vi "C State.vi"(0 "State":string, 1 "Front Leg PS":bool, 4 "Back Leg Up":bool, 5 "Mid Leg PS":bool, 6 "Back Leg PS":bool, 7 "Mid Leg Up":bool, 10 "Front Leg Up":bool, 11 "Back Claws Cmd":bool=TRUE, 13 "Front Claw Cmd":bool=TRUE) -> (20 "newState":string, 21 "Front Leg Cmd":enum16{"Down Closed", "Down Opened", "Up"}(ring), 22 "Drive Motor Enabled":bool=TRUE, 23 "Mid Leg Cmd":enum16{"Down Closed", "Down Opened", "Up"}(ring), 25 "Engage Back Leg":bool, 26 "Skids":bool)   [LabVIEW 2012]
uses:
  <vilib>/Rock Robotics/WPI/DriverStation/DriverStationLCD/WPI_DriverStationLCDLCDLine.ctl
  Begin/Global Variables.vi
panel:
  out "Error Text":string
  out "Console Msg":string
  out "Short Time Elapsed":bool caption="Time has Elapsed"
  out "Long Time Elapsed":bool
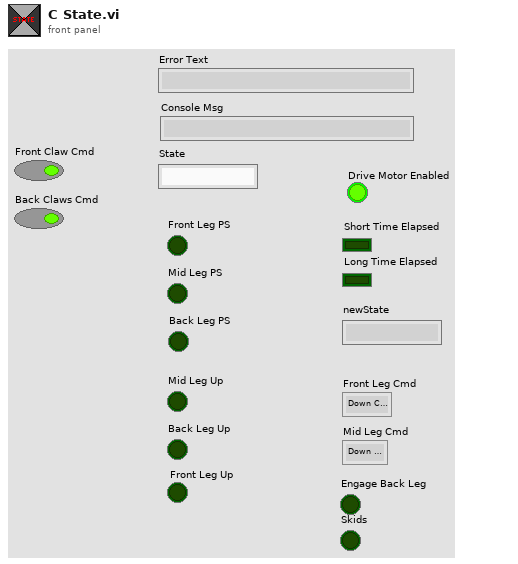
[diagram p1: front panel]
types:
  T1 = typedef "WPI_DriverStationLCDLCDLine.ctl" = enum16{"Main - Line 1", "User - Line 2", "User - Line 3", "User - Line 4", "User - Line 5", "User - Line 6"}
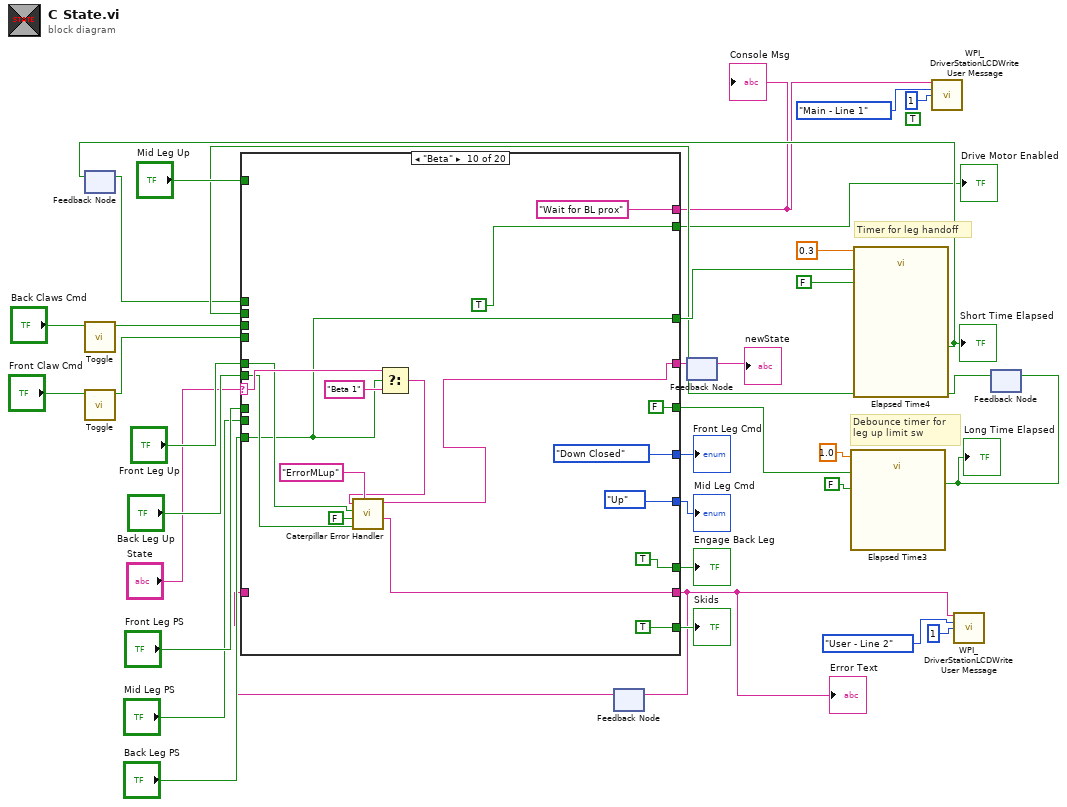
[diagram p0: block diagram]
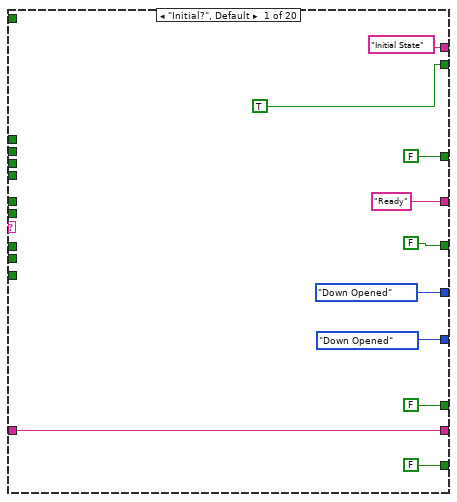
[diagram p2: hidden frame]
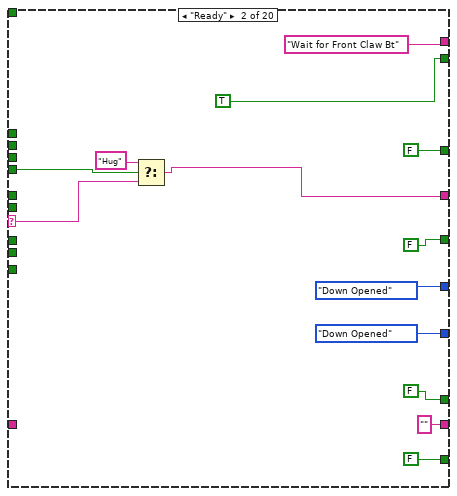
[diagram p3: hidden frame]
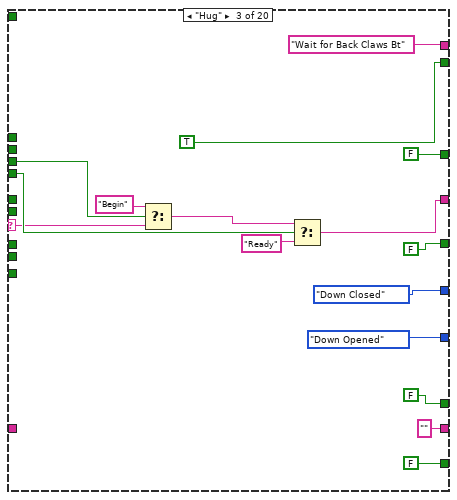
[diagram p4: hidden frame]
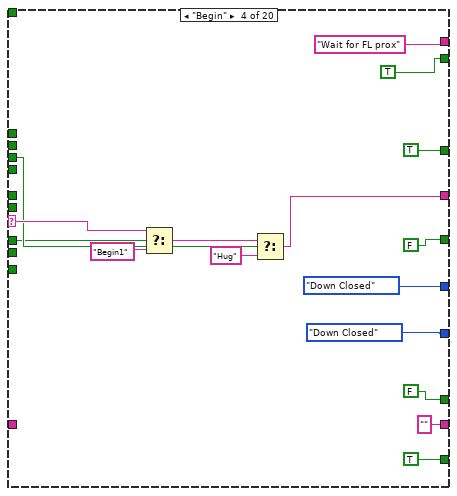
[diagram p5: hidden frame]
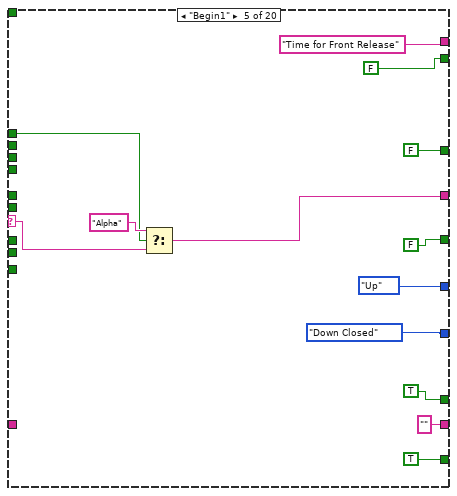
[diagram p6: hidden frame]
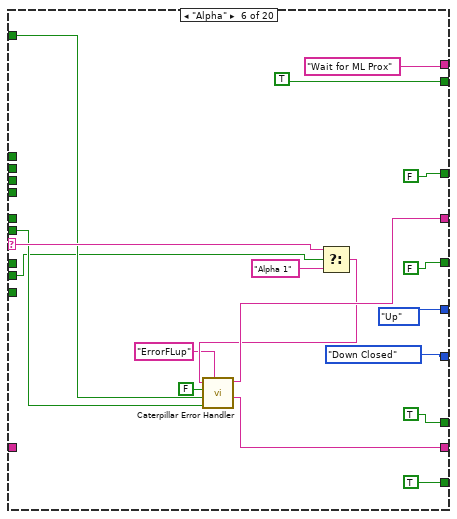
[diagram p7: hidden frame]
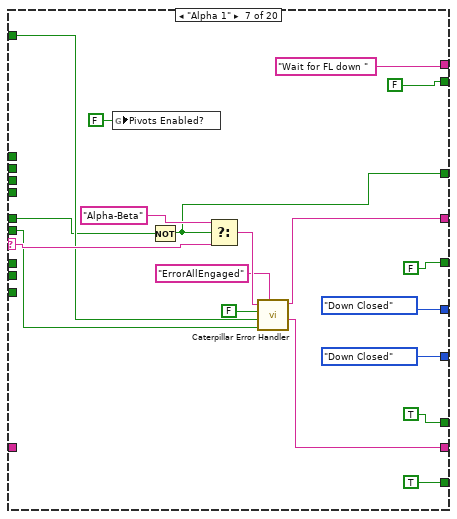
[diagram p8: hidden frame]
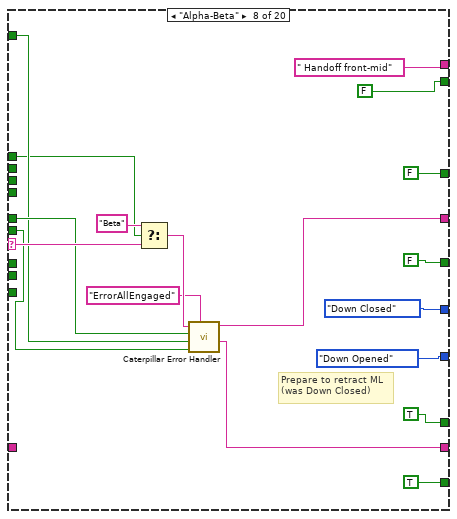
[diagram p9: hidden frame]
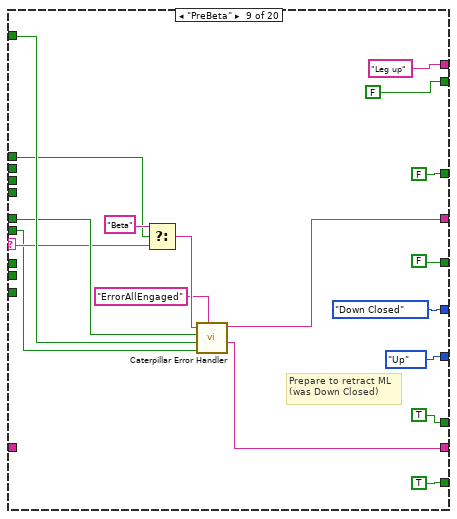
[diagram p10: hidden frame]
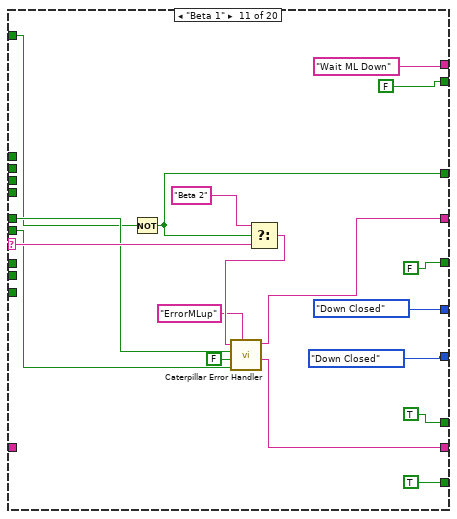
[diagram p11: hidden frame]
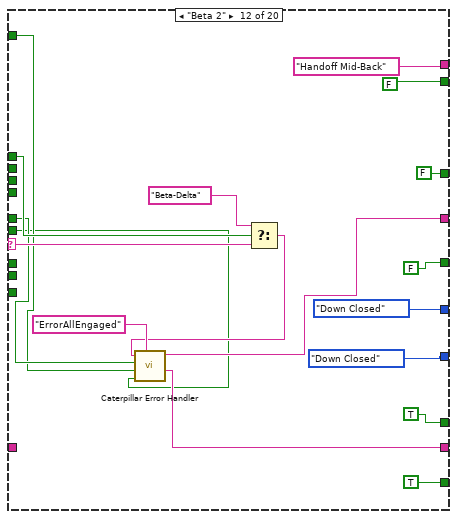
[diagram p12: hidden frame]
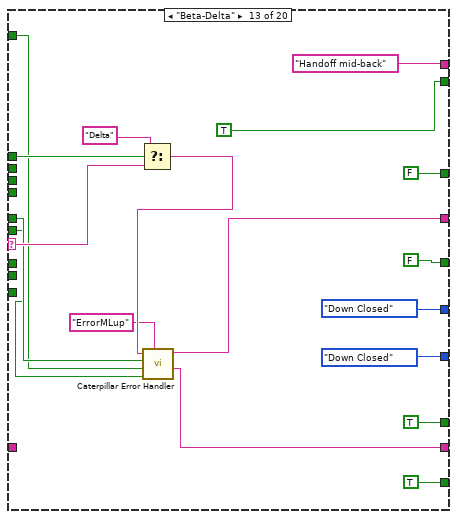
[diagram p13: hidden frame]
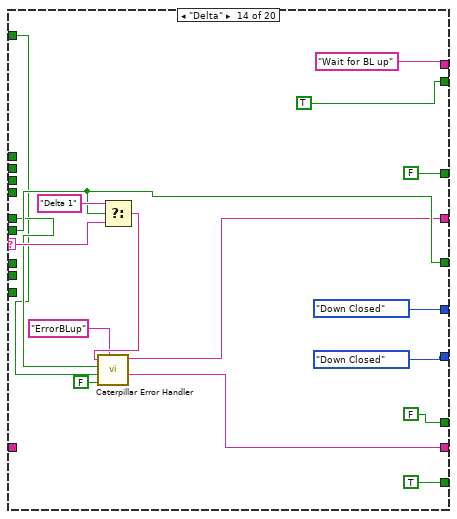
[diagram p14: hidden frame]
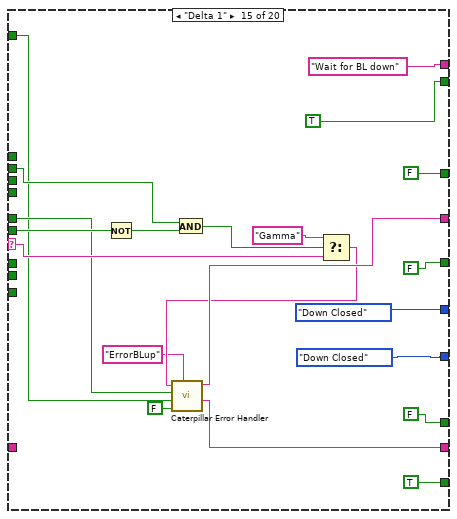
[diagram p15: hidden frame]
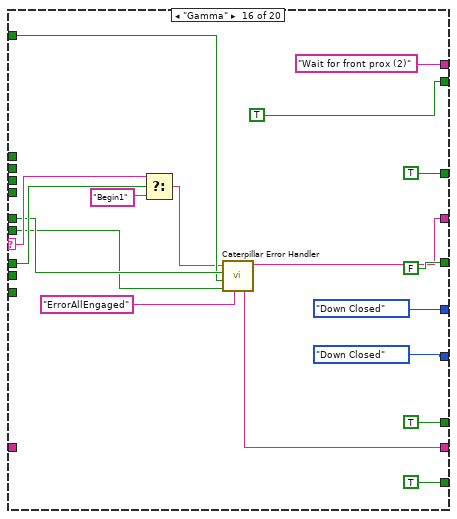
[diagram p16: hidden frame]
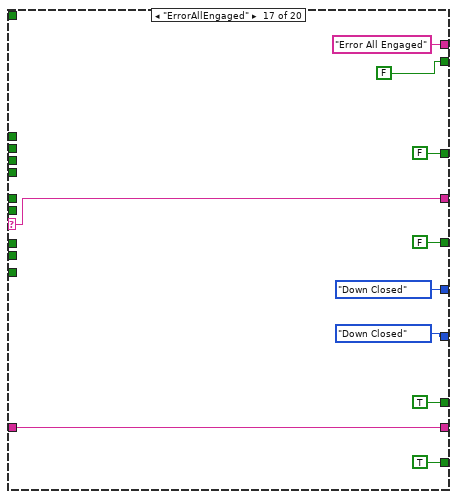
[diagram p17: hidden frame]
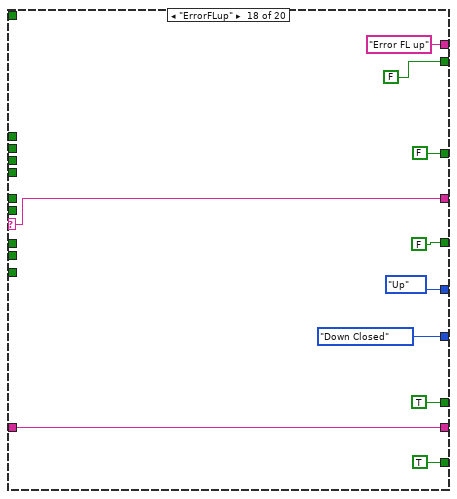
[diagram p18: hidden frame]
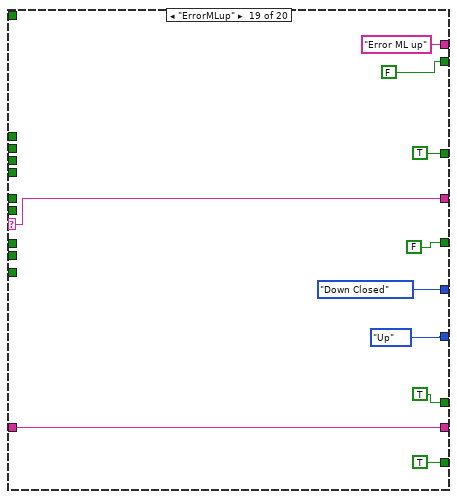
[diagram p19: hidden frame]
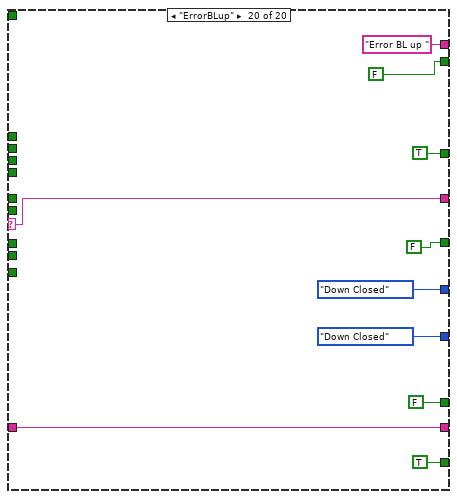
[diagram p20: hidden frame]
diagram:
  (unwired) TRUE ("clear line before write (T)")
  # "Timer for leg handoff"
  # "Debounce timer for \nleg up limit sw"
  n1 = feedback #1() -> (w17:bool)  [unwired: 1 in]
  n2 = call "Toggle.vi"("Boolean"="Back Claws Cmd") -> ("Toggled"=w15:bool)  [unwired: 10 in]
  n3 = call "Toggle.vi"("Boolean"="Front Claw Cmd") -> ("Toggled"=w24:bool)  [unwired: 10 in]
  n4 = feedback #2() -> (w6:string)  [unwired: 1 in]
  n5 = feedback #3() -> (→"newState":string)  [unwired: 1 in]
  n6 = feedback #4() -> (w23:bool)  [unwired: 1 in]
  n7 = case shown="\"Beta\"" "State" {
    selector: "State" -> [_ w56 w64 w84 w93 w119 w139 w156 w170 w186 w208 w226 w244 w260 w276 w301 w310 w320 w330 w340]
    tunnel: ["Ready" ("t") w49 w61 w78 w94 w111 w131 w150 w161 w183 w202 w217 w236 w254 w271 w293 w310 w320 w330 w340] -> w3
    tunnel: "Mid Leg PS" -> [_ _ _ _ _ w104 _ _ _ _ _ _ _ _ _ _ _ _ _ _]
    tunnel: "Front Leg PS" -> [_ _ _ w75 _ _ _ _ _ _ _ _ _ _ _ w300 _ _ _ _]
    tunnel: "Mid Leg Up" -> [_ _ _ _ _ w108 w130 w146 w173 _ w197 w214 w232 w250 w267 w289 _ _ _ _]
    tunnel: "Back Leg Up" -> [_ _ _ _ _ w107 w129 w145 w169 w179 w198 w213 w231 w259 w278 w290 _ _ _ _]
    tunnel: [FALSE FALSE ("clear line before write (T)") FALSE ("clear line before write (T)") FALSE ("clear line before write (T)") TRUE ("clear line before write (T)") TRUE ("clear line before write (T)") TRUE ("clear line before write (T)") TRUE ("clear line before write (T)") TRUE ("clear line before write (T)") TRUE ("clear line before write (T)") TRUE ("clear line before write (T)") TRUE ("clear line before write (T)") TRUE ("clear line before write (T)") FALSE ("clear line before write (T)") FALSE ("clear line before write (T)") TRUE ("clear line before write (T)") TRUE ("clear line before write (T)") TRUE ("clear line before write (T)") TRUE ("clear line before write (T)") FALSE ("clear line before write (T)")] -> w33
    tunnel: [FALSE FALSE FALSE TRUE TRUE TRUE TRUE TRUE TRUE TRUE TRUE TRUE TRUE TRUE TRUE TRUE TRUE TRUE TRUE TRUE] -> w32
    tunnel: w17 -> [_ _ _ _ w91 _ _ w141 w172 _ _ w220 w241 _ _ _ _ _ _ _]
    tunnel: [FALSE ("Time has Elapsed") FALSE ("Time has Elapsed") FALSE ("Time has Elapsed") TRUE ("Time has Elapsed") FALSE ("Time has Elapsed") FALSE ("Time has Elapsed") w124 FALSE ("Time has Elapsed") FALSE ("Time has Elapsed") w177 w203 FALSE ("Time has Elapsed") FALSE ("Time has Elapsed") FALSE ("Time has Elapsed") FALSE ("Time has Elapsed") TRUE ("Time has Elapsed") FALSE ("Time has Elapsed") FALSE ("Time has Elapsed") TRUE ("Time has Elapsed") TRUE ("Time has Elapsed")] -> w28
    tunnel: w23 -> [_ _ _ _ _ _ _ _ _ _ _ _ _ _ w282 _ _ _ _ _]
    tunnel: [FALSE FALSE FALSE ("Back Leg Up") FALSE FALSE FALSE FALSE FALSE FALSE FALSE ("Back Leg Up") FALSE FALSE FALSE w259 FALSE FALSE FALSE ("Back Leg Up") FALSE ("Back Leg Up") FALSE ("Back Leg Up") FALSE ("Back Leg Up")] -> w21
    tunnel: "Front Leg Up" -> [_ _ _ _ _ _ w122 w147 w171 w180 w199 w215 w233 w251 w268 w291 _ _ _ _]
    tunnel: [enum16{"Down Closed", "Down Opened", "Up"}."Down Opened" ("y") enum16{"Down Closed", "Down Opened", "Up"}."Down Opened" ("y") enum16{"Down Closed", "Down Opened", "Up"}."Down Closed" ("y") enum16{"Down Closed", "Down Opened", "Up"}."Down Closed" ("y") enum16{"Down Closed", "Down Opened", "Up"}."Up" ("y") enum16{"Down Closed", "Down Opened", "Up"}."Up" ("y") enum16{"Down Closed", "Down Opened", "Up"}."Down Closed" ("y") enum16{"Down Closed", "Down Opened", "Up"}."Down Closed" ("y") enum16{"Down Closed", "Down Opened", "Up"}."Down Closed" ("y") enum16{"Down Closed", "Down Opened", "Up"}."Down Closed" ("y") enum16{"Down Closed", "Down Opened", "Up"}."Down Closed" ("y") enum16{"Down Closed", "Down Opened", "Up"}."Down Closed" ("y") enum16{"Down Closed", "Down Opened", "Up"}."Down Closed" ("y") enum16{"Down Closed", "Down Opened", "Up"}."Down Closed" ("y") enum16{"Down Closed", "Down Opened", "Up"}."Down Closed" ("y") enum16{"Down Closed", "Down Opened", "Up"}."Down Closed" ("y") enum16{"Down Closed", "Down Opened", "Up"}."Down Closed" ("y") enum16{"Down Closed", "Down Opened", "Up"}."Up" ("y") enum16{"Down Closed", "Down Opened", "Up"}."Down Closed" ("y") enum16{"Down Closed", "Down Opened", "Up"}."Down Closed" ("y")] -> w26
    tunnel: w15 -> [_ _ w69 w83 _ _ _ _ _ _ _ _ _ _ _ _ _ _ _ _]
    tunnel: w24 -> [_ w46 w67 _ _ _ _ _ _ _ _ _ _ _ _ _ _ _ _ _]
    tunnel: "Back Leg PS" -> [_ _ _ _ _ _ _ _ _ w177 _ _ _ _ _ _ _ _ _ _]
    tunnel: [enum16{"Down Closed", "Down Opened", "Up"}."Down Opened" ("y") enum16{"Down Closed", "Down Opened", "Up"}."Down Opened" ("y") enum16{"Down Closed", "Down Opened", "Up"}."Down Opened" ("y") enum16{"Down Closed", "Down Opened", "Up"}."Down Closed" ("y") enum16{"Down Closed", "Down Opened", "Up"}."Down Closed" ("y") enum16{"Down Closed", "Down Opened", "Up"}."Down Closed" ("y") enum16{"Down Closed", "Down Opened", "Up"}."Down Closed" ("y") enum16{"Down Closed", "Down Opened", "Up"}."Down Opened" ("y") enum16{"Down Closed", "Down Opened", "Up"}."Up" ("y") enum16{"Down Closed", "Down Opened", "Up"}."Up" ("Mid Leg Cmd") enum16{"Down Closed", "Down Opened", "Up"}."Down Closed" ("y") enum16{"Down Closed", "Down Opened", "Up"}."Down Closed" ("y") enum16{"Down Closed", "Down Opened", "Up"}."Down Closed" ("y") enum16{"Down Closed", "Down Opened", "Up"}."Down Closed" ("y") enum16{"Down Closed", "Down Opened", "Up"}."Down Closed" ("y") enum16{"Down Closed", "Down Opened", "Up"}."Down Closed" ("y") enum16{"Down Closed", "Down Opened", "Up"}."Down Closed" ("y") enum16{"Down Closed", "Down Opened", "Up"}."Down Closed" ("y") enum16{"Down Closed", "Down Opened", "Up"}."Up" ("y") enum16{"Down Closed", "Down Opened", "Up"}."Down Closed" ("y")] -> w13
    tunnel: ["Initial State" ("line text") "Wait for Front Claw Bt" ("line text") "Wait for Back Claws Bt" ("line text") "Wait for FL prox" ("line text") "Time for Front Release" ("line text") "Wait for ML Prox" ("line text") "Wait for FL down " ("line text") " Handoff front-mid" ("line text") "Leg up" ("line text") "Wait for BL prox" ("line text") "Wait ML Down" ("line text") "Handoff Mid-Back" ("line text") "Handoff mid-back" ("line text") "Wait for BL up" ("line text") "Wait for BL down" ("line text") "Wait for front prox (2)" ("line text") "Error All Engaged" ("line text") "Error FL up" ("line text") "Error ML up" ("line text") "Error BL up " ("line text")] -> w10
    tunnel: [w37 "" ("Error Text") "" ("Error Text") "" ("Error Text") "" ("Error Text") w112 w126 w143 w168 w182 w196 w216 w235 w253 w272 w288 w305 w315 w325 w335] -> w5
    tunnel: w6 -> [w37 _ _ _ _ _ _ _ _ _ _ _ _ _ _ _ w305 w315 w325 w335]
    tunnel: [TRUE ("clear line before write (T)") TRUE ("clear line before write (T)") TRUE ("clear line before write (T)") TRUE ("clear line before write (T)") FALSE ("clear line before write (T)") TRUE ("clear line before write (T)") FALSE ("clear line before write (T)") FALSE ("clear line before write (T)") FALSE ("clear line before write (T)") TRUE ("clear line before write (T)") FALSE ("clear line before write (T)") FALSE ("clear line before write (T)") TRUE ("clear line before write (T)") TRUE ("clear line before write (T)") TRUE ("clear line before write (T)") TRUE ("clear line before write (T)") FALSE ("clear line before write (T)") FALSE ("clear line before write (T)") FALSE ("clear line before write (T)") FALSE ("clear line before write (T)")] -> w4
    frame "Initial?", Default {
    }
    frame "Ready" {
      n8 = Select(t="Hug", s=w46, f=w56) -> (s? t:f=w49:string)
    }
    frame "Hug" {
      n9 = Select(t="Begin", s=w69, f=w64) -> (s? t:f=w65:string)
      n10 = Select(t=w65, s=w67, f="Ready" ("t")) -> (s? t:f=w61:string)
    }
    frame "Begin" {
      n11 = Select(t=w84, s=w75, f="Begin1") -> (s? t:f=w82:string)
      n12 = Select(t=w82, s=w83, f="Hug") -> (s? t:f=w78:string)
    }
    frame "Begin1" {
      n13 = Select(t="Alpha" ("f"), s=w91, f=w93) -> (s? t:f=w94:string)
    }
    frame "Alpha" {
      n14 = Select(t=w119, s=w104, f="Alpha 1") -> (s? t:f=w110:string)
      n15 = call "Caterpillar Error Handler.vi"("Error State"="ErrorFLup", "Back Leg Up"=w107, "Mid Leg Up"=w108, "Front Leg Up"=FALSE, "state in"=w110) -> ("Error Text"=w112:string, "state out"=w111:string)  [unwired: 5 in]
    }
    frame "Alpha 1" {
      n16 = global write "Global Variables.vi" "Pivots Enabled?"(FALSE ("Pivots Enabled?")) -> ()
      n17 = Not(x=w122) -> (.not. x?=w124:bool)
      n18 = Select(t="Alpha-Beta" ("f"), s=w124, f=w139) -> (s? t:f=w132:string)
      n19 = call "Caterpillar Error Handler.vi"("Error State"="ErrorAllEngaged", "Back Leg Up"=w129, "Mid Leg Up"=w130, "Front Leg Up"=FALSE, "state in"=w132) -> ("Error Text"=w126:string, "state out"=w131:string)  [unwired: 5 in]
    }
    frame "Alpha-Beta" {
      # "Prepare to retract ML\n(was Down Closed)"
      n20 = Select(t="Beta" ("f"), s=w141, f=w156) -> (s? t:f=w151:string)
      n21 = call "Caterpillar Error Handler.vi"("Error State"="ErrorAllEngaged", "Back Leg Up"=w145, "Mid Leg Up"=w146, "Front Leg Up"=w147, "state in"=w151) -> ("Error Text"=w143:string, "state out"=w150:string)  [unwired: 5 in]
    }
    frame "PreBeta" {
      # "Prepare to retract ML\n(was Down Closed)"
      n22 = Select(t="Beta" ("f"), s=w172, f=w170) -> (s? t:f=w175:string)
      n23 = call "Caterpillar Error Handler.vi"("Error State"="ErrorAllEngaged", "Back Leg Up"=w169, "Mid Leg Up"=w173, "Front Leg Up"=w171, "state in"=w175) -> ("Error Text"=w168:string, "state out"=w161:string)  [unwired: 5 in]
    }
    frame "Beta" {
      n24 = Select(t=w186, s=w177, f="Beta 1") -> (s? t:f=w184:string)
      n25 = call "Caterpillar Error Handler.vi"("Error State"="ErrorMLup", "Back Leg Up"=w179, "Mid Leg Up"=FALSE, "Front Leg Up"=w180, "state in"=w184) -> ("Error Text"=w182:string, "state out"=w183:string)  [unwired: 5 in]
    }
    frame "Beta 1" {
      n26 = Not(x=w197) -> (.not. x?=w203:bool)
      n27 = Select(t="Beta 2" ("f"), s=w203, f=w208) -> (s? t:f=w201:string)
      n28 = call "Caterpillar Error Handler.vi"("Error State"="ErrorMLup", "Back Leg Up"=w198, "Mid Leg Up"=FALSE, "Front Leg Up"=w199, "state in"=w201) -> ("Error Text"=w196:string, "state out"=w202:string)  [unwired: 5 in]
    }
    frame "Beta 2" {
      n29 = Select(t="Beta-Delta" ("f"), s=w220, f=w226) -> (s? t:f=w218:string)
      n30 = call "Caterpillar Error Handler.vi"("Error State"="ErrorAllEngaged", "Back Leg Up"=w213, "Mid Leg Up"=w214, "Front Leg Up"=w215, "state in"=w218) -> ("Error Text"=w216:string, "state out"=w217:string)  [unwired: 5 in]
    }
    frame "Beta-Delta" {
      n31 = Select(t="Delta" ("f"), s=w241, f=w244) -> (s? t:f=w237:string)
      n32 = call "Caterpillar Error Handler.vi"("Error State"="ErrorMLup", "Back Leg Up"=w231, "Mid Leg Up"=w232, "Front Leg Up"=w233, "state in"=w237) -> ("Error Text"=w235:string, "state out"=w236:string)  [unwired: 5 in]
    }
    frame "Delta" {
      n33 = Select(t="Delta 1" ("f"), s=w259, f=w260) -> (s? t:f=w255:string)
      n34 = call "Caterpillar Error Handler.vi"("Error State"="ErrorBLup", "Back Leg Up"=FALSE, "Mid Leg Up"=w250, "Front Leg Up"=w251, "state in"=w255) -> ("Error Text"=w253:string, "state out"=w254:string)  [unwired: 5 in]
    }
    frame "Delta 1" {
      n35 = Not(x=w278) -> (.not. x?=w279:bool)
      n36 = And(x=w282, y=w279) -> (x .and. y?=w281:bool)
      n37 = Select(t="Gamma" ("f"), s=w281, f=w276) -> (s? t:f=w270:string)
      n38 = call "Caterpillar Error Handler.vi"("Error State"="ErrorBLup", "Back Leg Up"=FALSE, "Mid Leg Up"=w267, "Front Leg Up"=w268, "state in"=w270) -> ("Error Text"=w272:string, "state out"=w271:string)  [unwired: 5 in]
    }
    frame "Gamma" {
      n39 = Select(t=w301, s=w300, f="Begin1") -> (s? t:f=w286:string)
      n40 = call "Caterpillar Error Handler.vi"("Error State"="ErrorAllEngaged", "Back Leg Up"=w290, "Mid Leg Up"=w289, "Front Leg Up"=w291, "state in"=w286) -> ("Error Text"=w288:string, "state out"=w293:string)  [unwired: 5 in]
    }
    frame "ErrorAllEngaged" {
    }
    frame "ErrorFLup" {
    }
    frame "ErrorMLup" {
    }
    frame "ErrorBLup" {
    }
  }
  "Engage Back Leg" <- w33
  "Skids" <- w32
  "Front Leg Cmd" <- w26
  "Mid Leg Cmd" <- w13
  "Console Msg" <- w10
  "Error Text" <- w5
  "Drive Motor Enabled" <- w4
  n41 = feedback-in #2(w5) -> ()
  n42 = feedback-in #3(w3) -> ()
  n43 = call "Elapsed Time3"("Time Target (s)"=1.0, "Reset"=w21, "Auto Reset"=FALSE) -> ("Time has Elapsed"=w22:bool)  [unwired: 9 in, 7 out]
  "Long Time Elapsed" <- w22
  n44 = call "Elapsed Time4"("Time Target (s)"=0.3, "Reset"=w28, "Auto Reset"=FALSE) -> ("Time has Elapsed"=w18:bool)  [unwired: 9 in, 7 out]
  "Short Time Elapsed" <- w18
  n45 = feedback-in #1(w18) -> ()
  n46 = call <vilib>:"WPI_DriverStationLCDWrite User Message.vi"("line text"=w10, "line"=WPI_DriverStationLCDLCDLine."Main - Line 1", "starting column"=i8 1) -> ()  [unwired: 12 in, 1 out]
  n47 = call <vilib>:"WPI_DriverStationLCDWrite User Message.vi"("line text"=w5, "line"=WPI_DriverStationLCDLCDLine."User - Line 2", "starting column"=i8 1) -> ()  [unwired: 12 in, 1 out]
  n48 = feedback-in #4(w22) -> ()
